vi "Data update.vi"(0 "Lifter_motor in":refnum<class "Lifter_motor.lvclass">, 5 "ADC Distance":dbl, 7 "Step distance":dbl, 11 "error in (no error)":errorcluster) -> (4 "Lifter_motor out":refnum<class "Lifter_motor.lvclass">, 6 "New Data":bool, 15 "error out":errorcluster)   [LabVIEW 2019, in "Lifter_motor.lvclass"]
uses:
  Lifter_motor.lvclass
  Lifter_motor.lvclass/Lifter_motor.ctl
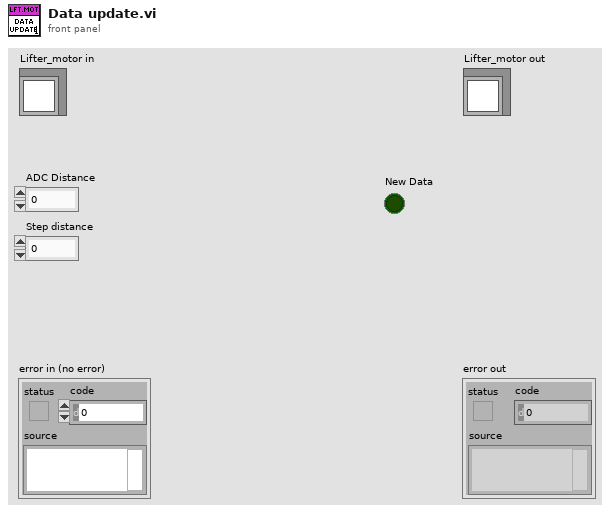
[diagram p1: front panel]
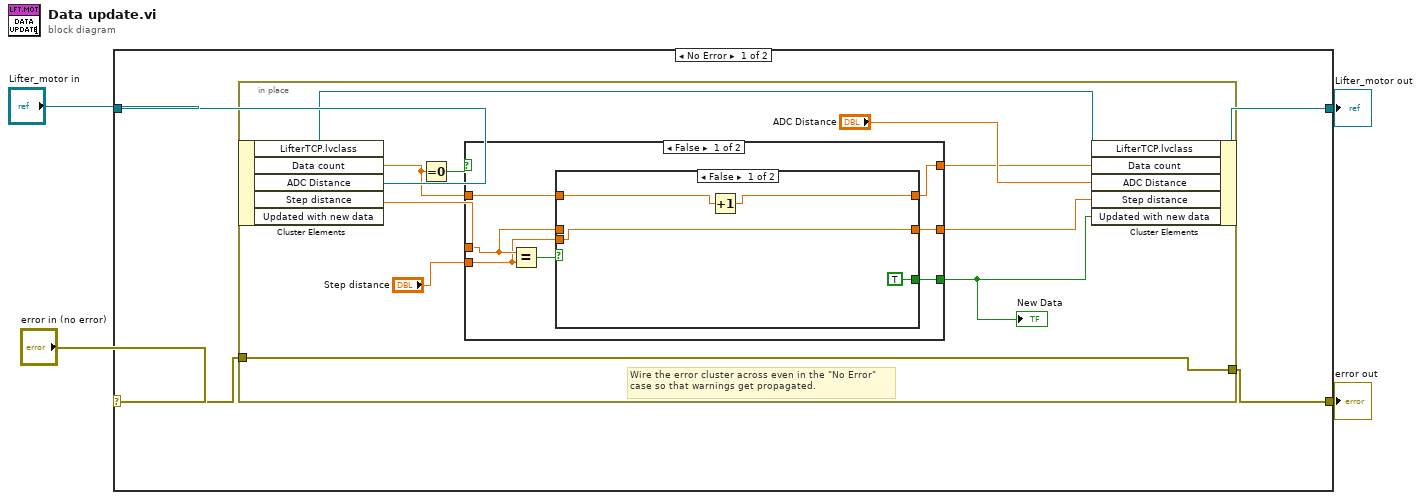
[diagram p0: block diagram]
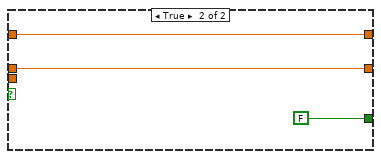
[diagram p2: hidden frame]
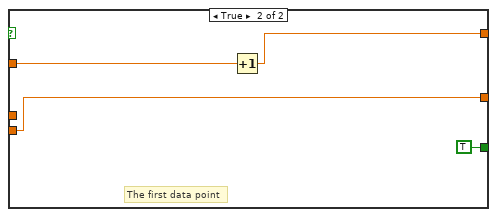
[diagram p3: hidden frame]
diagram:
  n1 = case shown="No Error" "error in (no error)" {
    selector: "error in (no error)" -> [w5 w38]
    tunnel: [w6 w38] -> w3
    tunnel: [w7 w37] -> w1
    tunnel: "Lifter_motor in" -> [w8 w37]
    frame No Error {
      n2 = in-place {
        in-place-border: [w10] -> w6
        in-place-border: w5 -> [w10]
        # "Wire the error cluster across even in the \"No Error\"\ncase so that warnings get propagated."
        n3 = in-place-cluster #1(w8) -> ("LifterTCP.lvclass"=w18:refnum<class "LifterTCP.lvclass">, "Data count"=w12:dbl, "Step distance"=w16:dbl)  [unwired: 2 out]
        n4 = Equal To 0?(x=w12) -> (x = 0?=w17:bool)
        n5 = case shown="False" w17 {
          tunnel: w16 -> [w23 _]
          tunnel: "Step distance" -> [w22 w36]
          tunnel: [w24 w36] -> w14
          tunnel: w12 -> [w21 w35]
          tunnel: [w20 w34] -> w11
          tunnel: [w19 TRUE ("New Data")] -> w9
          frame False {
            n6 = Equal?(x=w23, y=w22) -> (x = y?=w25:bool)
            n7 = case shown="False" w25 {
              tunnel: [w29 w32] -> w24
              tunnel: w23 -> [_ w32]
              tunnel: w22 -> [w29 _]
              tunnel: [w27 w30] -> w20
              tunnel: w21 -> [w26 w30]
              tunnel: [TRUE ("New Data") FALSE ("New Data")] -> w19
              frame False {
                n8 = Increment(x=w26) -> (x+1=w27:dbl)
              }
              frame True {
              }
            }
          }
          frame True {
            # "The first data point"
            n9 = Increment(x=w35) -> (x+1=w34:dbl)
          }
        }
        "New Data" <- w9
        n10 = in-place-cluster #1("LifterTCP.lvclass"=w18, "Data count"=w11, "ADC Distance"="ADC Distance", "Step distance"=w14, "Updated with new data"=w9) -> (w7:refnum<class "Lifter_motor.lvclass">)
      }
    }
    frame Error {
    }
  }
  "error out" <- w3
  "Lifter_motor out" <- w1
